vi "Stop Core.vi"(10 "final error code":i32, 11 "Topic In":refnum<class "Topic.lvclass">) -> (3 "Topic Out":refnum<class "Topic.lvclass">)   [LabVIEW 2017, in "Mediator.lvlib" / "Topic.lvclass"]
doc: "(<B>Filename</B>: Actor Framework.lvlib:Actor.lvclass:Stop Core.vi)\n\nDefines what the actor does before it stops. Use the <B>final error code</B> input to determine whether the actor shut down in response to an error.\n\nBy default, this method does nothing. A descendant class may override it to define behavior, such as shutting down any processes the actor initiated in its override of the Actor Core method."
uses:
  Topic.lvclass
  <vilib>/ActorFramework/Actor/Actor.lvclass
  gpm_packages/@cs/event-logger/Source/Composed Log/Types/Log Level.ctl
  gpm_packages/@cs/event-logger/Source/Composed Log/Composed Log.lvlib
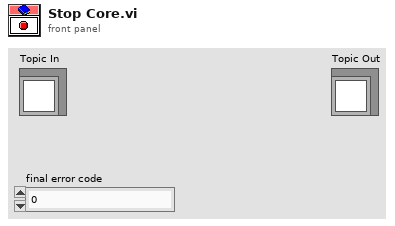
[diagram p1: front panel]
types:
  T1 = typedef "Composed Log.lvlib/Log Level.ctl" = enum16{"Debug", "Info", "Warning", "Error", "Critical"}
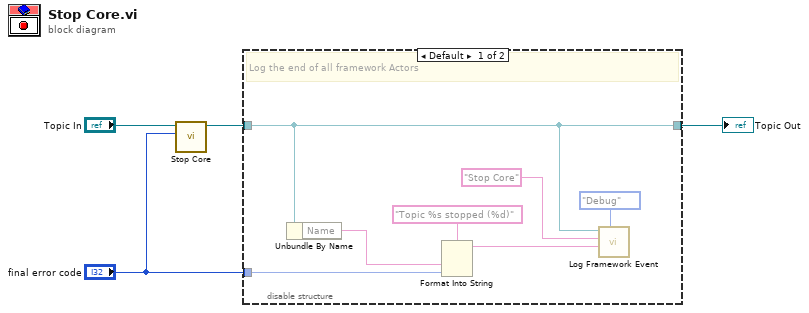
[diagram p0: block diagram]
diagram:
  n1 = call-parent "Stop Core.vi"("final error code"="final error code", "Actor in"="Topic In") -> ("Actor out"=w3:refnum<class "Topic.lvclass">)  [unwired: 9 in]
  n2 = disable-structure shown="Default" {
    disable-tunnel: w3 -> [w6 w12]
    disable-tunnel: [w6 w12] -> w2
    disable-tunnel: "final error code" -> [w10 _]
    frame condition #0 {
      # "Log the end of all framework Actors"
      n3 = Unbundle By Name(w6) -> ("Name"=w5:string)
      n4 = Format Into String(format string="Topic %s stopped (%d)", w5, w10) -> (resulting string=w8:string)  [unwired: 2 in, 1 out]
      n5 = call "Log Framework Event.vi"("Event Level (Debug)"=Log_Level."Debug" ("Event Level"), "Data To Log"=w8, "Caller Info (\"\")"="Stop Core" ("Caller Info (\"\")"), "Topic In"=w6) -> ()  [unwired: 7 in, 1 out]
    }
    frame condition #1 (active) {
      # "Remove all logging from this method at compile time"
    }
  }
  "Topic Out" <- w2
